vi "Win_Touch.vi"(8 "error in (no error)":errorcluster, 11 "TouchXY":string) -> (0 "error out":errorcluster)   [LabVIEW 2025]
uses:
  Controls/TouchXY.ctl
  07b9a5a2-ecad-467c-a685-a203eddfa678.vi
  35da1dd9-0731-4e8b-97e7-5043d3958051.vi
  752d6ef3-87c6-4ef9-a639-d3e4bb901061.vi
  018a0e81-23d2-474a-a46f-ccfe828a7f0e.vi
  0a09c8df-c8d5-4fdf-ba9c-67257bbb9353.vi
  user32.dll
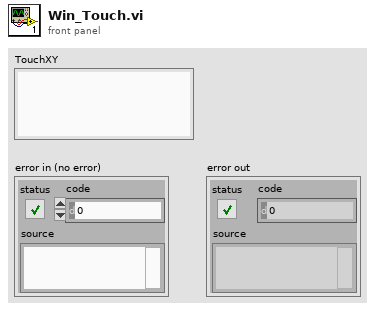
[diagram p1: front panel]
types:
  T1 = typedef "TouchXY.ctl" = cluster{"Win Name":string, "TouchCoord":cluster{"x":sgl, "y":sgl}}
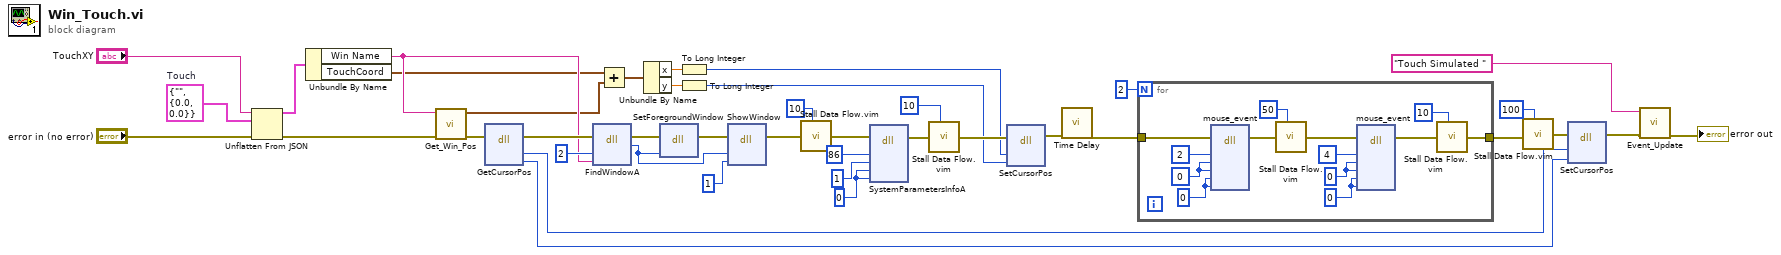
[diagram p0: block diagram]
diagram:
  w12 = T1 {"Win Name"="", "TouchCoord"={"x"=0.0, "y"=0.0}}  # Touch
  w33 = 0
  n1 = Unflatten From JSON(JSON string="TouchXY", type and defaults=w12, error in (no error)="error in (no error)") -> (value=w9:T1, error out=w8:errorcluster)  [unwired: 4 in]
  n2 = Unbundle By Name(w9) -> ("Win Name"=w6:string, "TouchCoord"=w2:cluster{"x":sgl, "y":sgl})
  n3 = call "Get_Win_Pos.vi"("error in (no error)"=w8, "Win Name"=w6) -> ("error out"=w7:errorcluster, "Win_Position"=w1:cluster{"x":sgl, "y":sgl})  [unwired: 8 in]
  n4 = dll-call lib="user32.dll" fn="GetCursorPos"(error in=w7) -> (error out=w18:errorcluster, "x"=w17:i32, "y"=w16:i32)  [unwired: 3 in, 3 out]
  n5 = dll-call lib="user32.dll" fn="FindWindowA"(error in=w18, "arg1"=2, "arg2"=w6) -> (error out=w23:errorcluster, "return type"=w21:i32)  [unwired: 3 in, 2 out]
  n6 = Add(x=w2, y=w1) -> (x+y=w36:cluster{"x":sgl, "y":sgl})
  n7 = Unbundle By Name(w36) -> ("x"=w39:sgl, "y"=w38:sgl)
  n8 = dll-call lib="user32.dll" fn="SetForegroundWindow"(error in=w23, "arg1"=w21) -> (error out=w22:errorcluster)  [unwired: 3 in, 2 out]
  n9 = To Long Integer(number=w39) -> (32bit integer=w20:i32)
  n10 = To Long Integer(number=w38) -> (32bit integer=w19:i32)
  n11 = dll-call lib="user32.dll" fn="ShowWindow"(error in=w22, "arg1"=w21, "arg2"=1) -> (error out=w26:errorcluster)  [unwired: 4 in, 2 out]
  n12 = call "Stall Data Flow.vim"("value in"=w26, "milliseconds to wait"=u32 10) -> ("value out"=w27:errorcluster)  [unwired: 1 out]
  n13 = dll-call lib="user32.dll" fn="SystemParametersInfoA" ("Terminate power-off mode")(error in=w27, "uiAction"=u32 86 ("SPI_GETPOWEROFFACTIVE"), "uiParam"=u32 1 ("Off"), "pvParam"=w33, "fWinIni"=w33) -> (error out=w31:errorcluster)  [unwired: 7 in, 1 out]
  n14 = call "Stall Data Flow.vim"("value in"=w31, "milliseconds to wait"=u32 10) -> ("value out"=w37:errorcluster)  [unwired: 1 out]
  n15 = dll-call lib="User32.dll" fn="SetCursorPos"(error in=w37, w20, w19) -> (error out=w40:errorcluster)  [unwired: 5 in, 1 out]
  n16 = call "Time Delay"("error in (no error)"=w40) -> ("error out"=w34:errorcluster)  [unwired: 10 in]
  n17 = for {
    N: 2 ("Count") -> [_]
    tunnel: w34 -> [w52]
    tunnel: [w42] -> w14
    w50 = 0 ("dwExtraInfo")
    w51 = u32 0 ("dwExtraInfo")
    w53 = 0 ("dwExtraInfo")
    w49 = u32 0 ("dwExtraInfo")
    n18 = dll-call lib="user32.dll" fn="mouse_event" label="Click"(error in=w52, "dwFlags"=2, "dx"=w53, "dy"=w53, "dwData"=w49, "dwExtraInfo"=w49) -> (error out=w44:errorcluster)  [unwired: 8 in, 1 out]
    n19 = call "Stall Data Flow.vim"("value in"=w44, "milliseconds to wait"=u32 50) -> ("value out"=w46:errorcluster)  [unwired: 1 out]
    n20 = dll-call lib="user32.dll" fn="mouse_event" label="Release"(error in=w46, "dwFlags"=4, "dx"=w50, "dy"=w50, "dwData"=w51, "dwExtraInfo"=w51) -> (error out=w43:errorcluster)  [unwired: 8 in, 1 out]
    n21 = call "Stall Data Flow.vim"("value in"=w43, "milliseconds to wait"=u32 10) -> ("value out"=w42:errorcluster)  [unwired: 1 out]
  }
  n22 = call "Stall Data Flow.vim"("value in"=w14, "milliseconds to wait"=u32 100) -> ("value out"=w13:errorcluster)  [unwired: 1 out]
  n23 = dll-call lib="User32.dll" fn="SetCursorPos"(error in=w13, w17, w16) -> (error out=w5:errorcluster)  [unwired: 5 in, 1 out]
  n24 = call "Event_Update.vi"("Error In"=w5, "Event"="Touch Simulated ") -> ("Error Out"=→"error out":errorcluster)  [unwired: 9 in]
